vi "Reserve Sessions with Observer.vi"(6 "timeout (ms)":i32, 7 "reservation observer":refnum<class "IReservation Observer.lvclass">, 8 "error in":errorcluster, 9 "instrument type id":string, 10 "pin or relay names":string[](array[string]), 11 "pin map context":T1) -> (0 "error out":errorcluster, 3 "session reservation out":refnum<class "Session Reservation.lvclass">)   [LabVIEW 2021, in "NI Session Management V1 Client.lvlib" / "Session Reservation.lvclass"]
doc: "Reserves session(s) based on the provided instrument type and pin or its group information."
uses:
  Session Reservation.lvclass
  Session Reservation.lvclass/Session Reservation.ctl
  gRPC/Generated APIs/ni/measurementlink/sessionmanagement/v1/RPC Messages/ni_measurementlink_sessionmanagement_v1_ReserveSessionsRequest.ctl
  gRPC/Generated APIs/ni/measurementlink/sessionmanagement/v1/ni.measurementlink.sessionmanagement.v1.api.lvlib
  gRPC/Generated APIs/ni/measurementlink/sessionmanagement/v1/RPC Messages/ni_measurementlink_PinMapContext.ctl
  gRPC/Generated APIs/ni/measurementlink/sessionmanagement/v1/RPC Messages/ni_measurementlink_sessionmanagement_v1_ReserveSessionsRequest_AnnotationsEntry.ctl
  IReservation Observer/IReservation Observer.lvclass
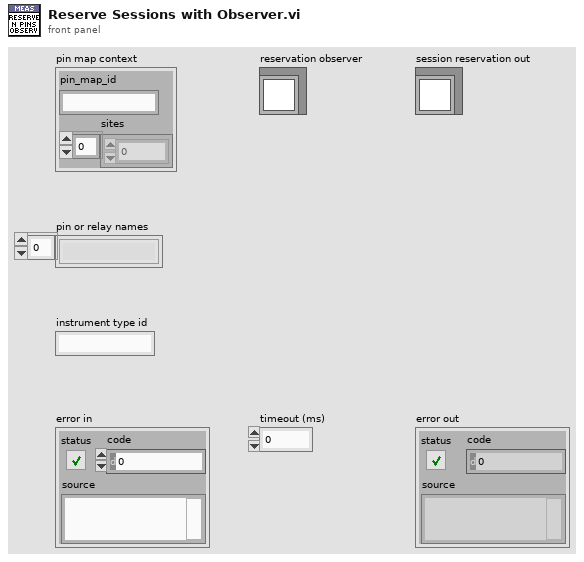
[diagram p1: front panel]
types:
  T1 = typedef "ni.measurementlink.sessionmanagement.v1.api.lvlib/ni_measurementlink_PinMapContext.ctl" = cluster{"pin_map_id":string, "sites":i32[]}
  T2 = typedef "ni.measurementlink.sessionmanagement.v1.api.lvlib/ni_measurementlink_sessionmanagement_v1_ReserveSessionsRequest.ctl" = cluster{"pin_map_context":T1, "pin_or_relay_names":string[], "instrument_type_id":string, "timeout_in_milliseconds":i32, "annotations":T3[]}
  T3 = typedef "ni.measurementlink.sessionmanagement.v1.api.lvlib/ni_measurementlink_sessionmanagement_v1_ReserveSessionsRequest_AnnotationsEntry.ctl" = cluster{"key":string, "value":string}
  T4 = typedef "ni.measurementlink.sessionmanagement.v1.api.lvlib/ni_measurementlink_sessionmanagement_v1_ReserveSessionsResponse.ctl" = cluster{"sessions":T5[], "multiplexer_sessions":T9[], "group_mappings":T11[]}
  T5 = typedef "ni.measurementlink.sessionmanagement.v1.api.lvlib/ni_measurementlink_sessionmanagement_v1_SessionInformation.ctl" = cluster{"session":T6, "resource_name":string, "channel_list":string, "instrument_type_id":string, "session_exists":bool, "session_reserved":bool, "channel_mappings":T7[], "annotations":T8[]}
  T6 = typedef "ni.measurementlink.sessionmanagement.v1.api.lvlib/nidevice_grpc_Session.ctl" = cluster{"name":string}
  T7 = typedef "ni.measurementlink.sessionmanagement.v1.api.lvlib/ni_measurementlink_sessionmanagement_v1_ChannelMapping.ctl" = cluster{"pin_or_relay_name":string, "site":i32, "channel":string, "multiplexer_resource_name":string, "multiplexer_route":string}
  T8 = typedef "ni.measurementlink.sessionmanagement.v1.api.lvlib/ni_measurementlink_sessionmanagement_v1_SessionInformation_AnnotationsEntry.ctl" = cluster{"key":string, "value":string}
  T9 = typedef "ni.measurementlink.sessionmanagement.v1.api.lvlib/ni_measurementlink_sessionmanagement_v1_MultiplexerSessionInformation.ctl" = cluster{"session":T6, "resource_name":string, "multiplexer_type_id":string, "session_exists":bool, "annotations":T10[]}
  T10 = typedef "ni.measurementlink.sessionmanagement.v1.api.lvlib/ni_measurementlink_sessionmanagement_v1_MultiplexerSessionInformation_AnnotationsEntry.ctl" = cluster{"key":string, "value":string}
  T11 = typedef "ni.measurementlink.sessionmanagement.v1.api.lvlib/ni_measurementlink_sessionmanagement_v1_ReserveSessionsResponse_GroupMappingsEntry.ctl" = cluster{"key":string, "value":T12}
  T12 = typedef "ni.measurementlink.sessionmanagement.v1.api.lvlib/ni_measurementlink_sessionmanagement_v1_ResolvedPinsOrRelays.ctl" = cluster{"pin_or_relay_names":string[]}
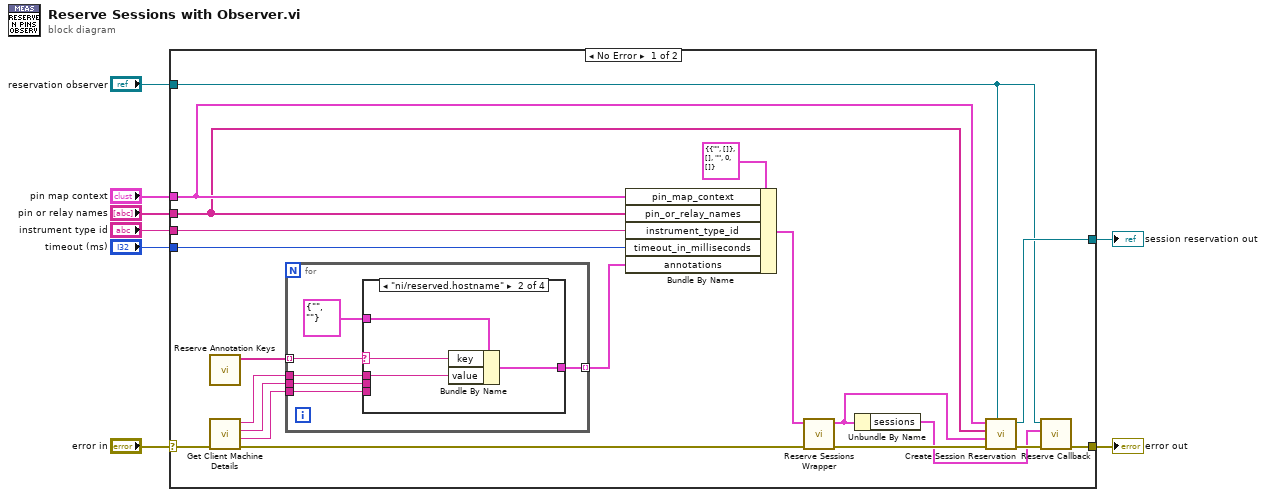
[diagram p0: block diagram]
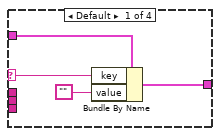
[diagram p2: hidden frame]
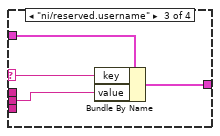
[diagram p3: hidden frame]
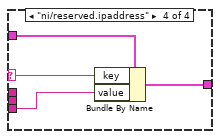
[diagram p4: hidden frame]
diagram:
  n1 = case shown="No Error" "error in" {
    selector: "error in" -> [w12 w51]
    tunnel: "instrument type id" -> [w27 _]
    tunnel: "pin or relay names" -> [w22 _]
    tunnel: "timeout (ms)" -> [w26 _]
    tunnel: "pin map context" -> [w23 _]
    tunnel: [w20 w51] -> w4
    tunnel: [w24 _] -> w3
    tunnel: "reservation observer" -> [w19 _]
    frame No Error {
      n2 = call "Reserve Annotation Keys.vi"() -> ("reserve annotation keys"=w16:string[])  [unwired: 11 in]
      n3 = call "Get Client Machine Details.vi"("error in"=w12) -> ("error out"=w11:errorcluster, "ip address"=w13:string, "username"=w14:string, "hostname"=w15:string)  [unwired: 7 in]
      n4 = for {
        tunnel: [w34] -> w10 mode=indexing
        tunnel: w16 -> [w33] mode=indexing
        tunnel: w13 -> [w32]
        tunnel: w14 -> [w31]
        tunnel: w15 -> [w30]
        n5 = case shown="\"ni/reserved.hostname\"" w33 {
          selector: w33 -> [w38 w41 w45 w49]
          tunnel: T3 {"key"="", "value"=""} ("ni_measurementlink_sessionmanagement_v1_ReserveSessionsRequest_AnnotationsEntry") -> [w35 w42 w46 w50]
          tunnel: [w36 w40 w44 w48] -> w34
          tunnel: w32 -> [_ _ _ w47]
          tunnel: w31 -> [_ _ w43 _]
          tunnel: w30 -> [_ w39 _ _]
          frame Default {
            n6 = Bundle By Name(cluster=w35, "key"=w38, "value"="") -> (w36:T3)
          }
          frame "ni/reserved.hostname" {
            n7 = Bundle By Name(cluster=w42, "key"=w41, "value"=w39) -> (w40:T3)
          }
          frame "ni/reserved.username" {
            n8 = Bundle By Name(cluster=w46, "key"=w45, "value"=w43) -> (w44:T3)
          }
          frame "ni/reserved.ipaddress" {
            n9 = Bundle By Name(cluster=w50, "key"=w49, "value"=w47) -> (w48:T3)
          }
        }
      }
      n10 = Bundle By Name(cluster=T2 {"pin_map_context"={"pin_map_id"="", "sites"=[]}, "pin_or_relay_names"=[], "instrument_type_id"="", "timeout_in_milliseconds"=0, "annotations"=[]} ("Request Data"), "pin_map_context"=w23, "pin_or_relay_names"=w22, "instrument_type_id"=w27, "timeout_in_milliseconds"=w26, "annotations"=w10) -> (w17:T2)
      n11 = call "Reserve Sessions Wrapper.vi"("error in"=w11, "request data"=w17) -> ("error out"=w25:errorcluster, "response data"=w9:T4)  [unwired: 8 in]
      n12 = Unbundle By Name(w9) -> ("sessions"=w18:T5[])
      n13 = call "Create Session Reservation.vi"("reservation observer"=w19, "error in"=w25, "session reservation response"=w9, "pin or relay names"=w22, "pin map context"=w23) -> ("error out"=w21:errorcluster, "session reservation out"=w24:refnum<class "Session Reservation.lvclass">)  [unwired: 5 in]
      n14 = call-dynamic "Reserve Callback.vi"("error in"=w21, "session infos"=w18, "reservation observer in"=w19) -> ("error out"=w20:errorcluster)  [unwired: 7 in, 1 out]
    }
    frame Error {
    }
  }
  "session reservation out" <- w3
  "error out" <- w4
